vi "getIntValue.vi"(8 "error in (no error)":errorcluster, 11 "INumber in":refnum<class "INumber.lvclass">) -> (0 "error out":errorcluster, 2 "Int Value out":i64, 3 "INumber out":refnum<class "INumber.lvclass">)   [LabVIEW 2022 SP3, in "openDAQ.lvlib" / "daqCoreTypes.lvlib" / "INumber.lvclass"]
uses:
  <instrlib>/openDAQ/Public/Classes/daqCoreTypes/INumber/INumber.lvclass
  <instrlib>/openDAQ/Public/Classes/daqCoreTypes/INumber/INumber.lvclass/INumber.ctl
  <instrlib>/openDAQ/Binaries/Windows/x86/copendaq32.dll
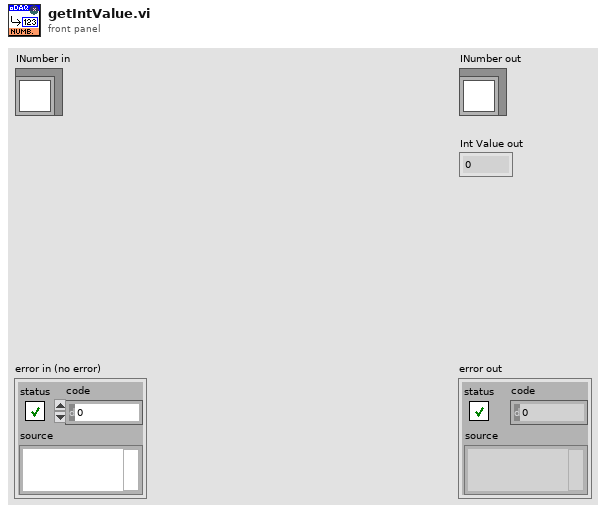
[diagram p1: front panel]
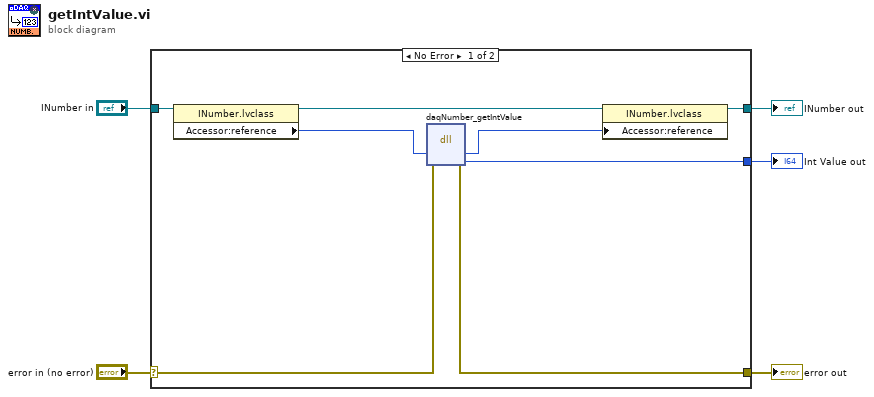
[diagram p0: block diagram]
diagram:
  n1 = case shown="No Error" "error in (no error)" {
    selector: "error in (no error)" -> [w12 w15]
    tunnel: [w11 w15] -> w4
    tunnel: [w8 w14] -> w3
    tunnel: "INumber in" -> [w13 w14]
    tunnel: [w7 _] -> w2
    frame No Error {
      n2 = property class="INumber.lvclass"(reference=w13) -> (reference out=w6:refnum<class "INumber.lvclass">, "Accessor:reference"=w10:i64)  [unwired: 1 in, 1 out]
      n3 = dll-call lib="C:/Program Files (x86)/National Instruments/LabVIEW 2022/instr.lib/openDAQ/Binaries/Windows/x86/copendaq*.*" fn="daqNumber_getIntValue"(error in=w12, "number"=w10) -> (error out=w11:errorcluster, "number"=w9:i64, "intValue"=w7:i64)  [unwired: 4 in, 1 out]
      n4 = property class="INumber.lvclass"(reference=w6, "Accessor:reference"=w9) -> (reference out=w8:refnum<class "INumber.lvclass">)  [unwired: 1 in, 1 out]
    }
    frame Error {
    }
  }
  "error out" <- w4
  "INumber out" <- w3
  "Int Value out" <- w2
